vi "Database Module.vi"(8 "error in":errorcluster) -> (0 "error out":errorcluster)   [LabVIEW 2018, in "Database.lvlib"]
doc: "This is the top level of the database module (a free running module of the Car Wash simulator). \n\nIt is closed using a user event. It communicates with the other modules using a queue based API which has comms modules that can be swapped if required."
uses:
  Database.lvlib
  Private Controls/Module Data Cluster.ctl
  Private Controls/Module Action.ctl
  <vilib>/addons/database/_DB Variant To Data/Database Variant To Data.xnode
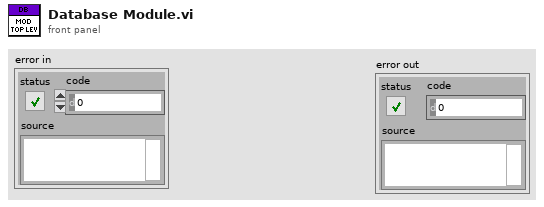
[diagram p1: front panel]
types:
  T1 = cluster{"Step Duration":string, "Station":string, "Wash Step":string}
  T2 = typedef "Database.lvlib/Module Data Cluster.ctl" = cluster{"Variant":variant, "action":T3}
  T3 = typedef "Database.lvlib/Module Action.ctl" = enum16{"error", "exit", "init", "Read Database Record", "Query Timing", "Update record", "Insert Record", "Release Connection"}
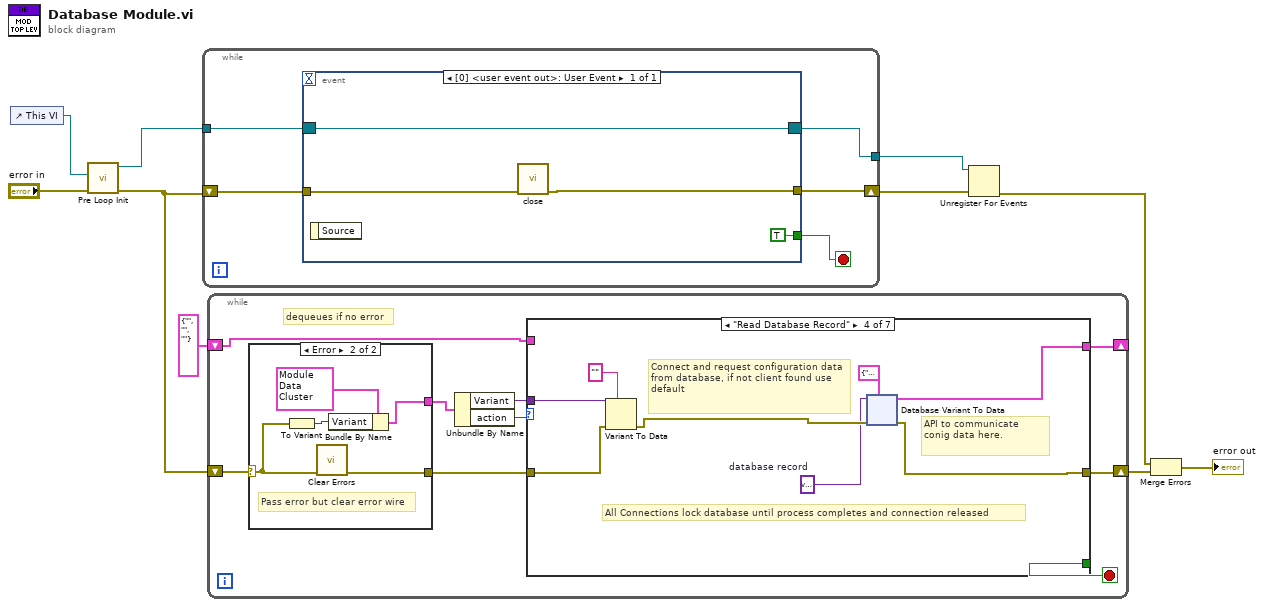
[diagram p0: block diagram]
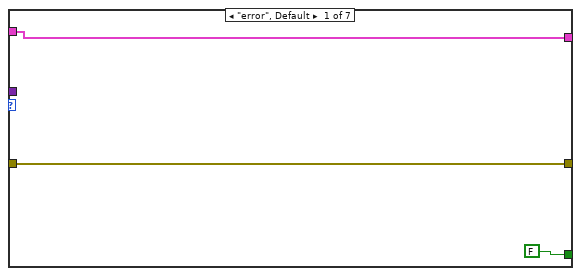
[diagram p2: hidden frame]
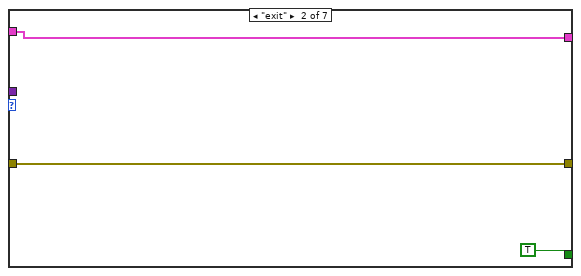
[diagram p3: hidden frame]
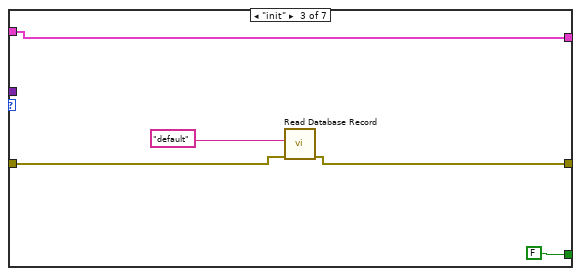
[diagram p4: hidden frame]
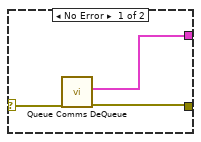
[diagram p8: hidden frame]
diagram:
  n1 = control-ref of="This VI"() -> (w10:refnum<vi>)
  n2 = call "Pre Loop Init.vi"("error in"="error in", "Ref In"=w10) -> ("error out"=w7:errorcluster, "Event Registration Refnum"=w9:refnum<event-registration>)  [unwired: 8 in]
  n3 = while {
    shift-right: [w14] -> w6
    shift-left: w7 -> [w15]
    tunnel: w9 -> [w13]
    tunnel: [w11] -> w5
    stop <- w12 stop-if-true
    n4 = event shown="[0] <user event out>: User Event" {
      selector: w13 -> [w16]
      dyn-events: [w16] -> w11
      timeout: _ -> [_]
      tunnel: w15 -> [w19]
      tunnel: [w18] -> w14
      tunnel: [TRUE] -> w12
      event User Event {
        n5 = event-data() -> ()  [unwired: 1 in, 1 out]
        n6 = call "close.vi"("error in"=w19) -> ("error out"=w18:errorcluster)  [unwired: 10 in]
      }
    }
  }
  n7 = while {
    shift-right: [w24] -> w4
    shift-left: w7 -> [w28]
    shift-right: [w21] -> _
    shift-left: T1 {"Step Duration"="", "Station"="", "Wash Step"=""} ("data") -> [w20]
    stop <- w22 stop-if-true
    # "dequeues if no error"
    n8 = case shown="Error" w28 {
      selector: w28 -> [w91 w96]
      tunnel: [w90 w92] -> w27
      tunnel: [w89 w95] -> w23
      frame No Error {
        n9 = call "Queue Comms DeQueue.vi"("error in"=w91) -> ("error out"=w89:errorcluster, "element"=w90:T2)  [unwired: 9 in]
      }
      frame Error {
        # "Pass error but clear error wire"
        n10 = To Variant(anything=w96) -> (Variant=w93:variant)
        n11 = call <vilib>:"Clear Errors.vi"("error in (no error)"=w96) -> ("error out"=w95:errorcluster)  [unwired: 5 in, 1 out]
        n12 = Bundle By Name(cluster=T2 {"Variant"=variant, "action"=enum."error"} ("element"), "Variant"=w93) -> (w92:T2)
      }
    }
    n13 = Unbundle By Name(w27) -> ("Variant"=w25:variant, "action"=w26:T3)
    n14 = case shown="\"Read Database Record\"" w26 {
      tunnel: w25 -> [_ _ _ w47 _ _ _]
      tunnel: [w31 w34 w37 w40 w84 w86 w88] -> w24
      tunnel: w23 -> [w31 w34 w38 w43 w84 w86 w88]
      tunnel: [FALSE TRUE FALSE _ _ _ _] -> w22
      tunnel: [w29 w32 w35 w44 w83 w85 w87] -> w21
      tunnel: w20 -> [w29 w32 w35 _ w83 w85 w87]
      frame "error", Default {
      }
      frame "exit" {
      }
      frame "init" {
        n15 = call "Read Database Record.vi"("error in"=w38, "data"="default" ("client")) -> ("error out"=w37:errorcluster)  [unwired: 9 in]
      }
      frame "Read Database Record" {
        w41 = variant  # database record
        # "API to communicate conig data here."
        # "All Connections lock database until process completes and connection released"
        # "Connect and request configuration data from database, if not client found use default"
        n16 = Variant To Data(error in=w43, type="" ("client"), Variant=w47) -> (error out=w42:errorcluster)  [unwired: 1 out]
        n17 = xnode "Database Variant To Data"("database variant"=w41, "error in (no error)"=w42, "type"=T1 {"Step Duration"="", "Station"="", "Wash Step"=""} ("Database Record")) -> ("data"=w44:T1, "error out"=w40:errorcluster)
      }
      frame "Release Connection" {
        # "[Covers : SD7]"
        # "at the end of every connection to the database, release the connection"
      }
      frame "Update record" {
      }
      frame "Insert Record" {
      }
    }
  }
  n18 = Unregister For Events(event registration refnum=w5, error in=w6) -> (error out=w2:errorcluster)
  n19 = Merge Errors(w2, w4) -> (→"error out":errorcluster)
